vi "Plot Attributes.vi"(8 "error in (no error)":errorcluster, 10 "feature names":string[](array[string])=["feature1", "feature2", "feature3", "feature4"], 11 "appended array":refnum<vi>[](array[refnum])) -> (0 "error in (no error)":errorcluster)   [LabVIEW 2017, in "MachineLearning.lvlib"]
doc: "Replaces the plot names in the plot legend with the feature names for one or multiple waveform graphs."
uses:
  MachineLearning.lvlib
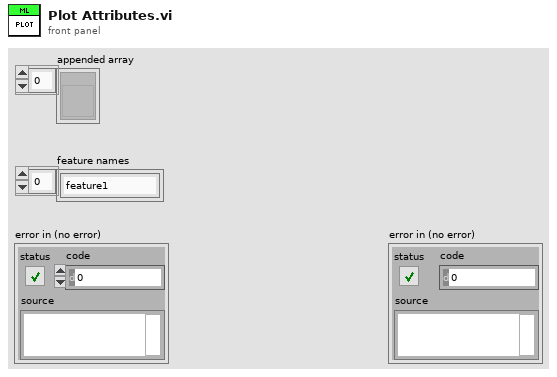
[diagram p1: front panel]
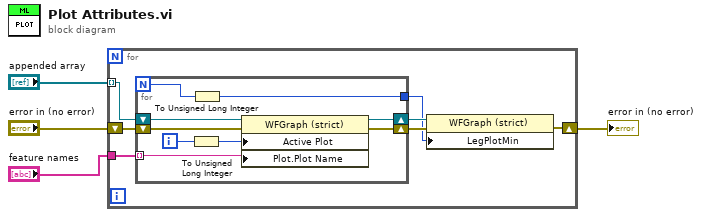
[diagram p0: block diagram]
diagram:
  n1 = for {
    tunnel: "appended array" -> [w7] mode=indexing
    tunnel: "feature names" -> [w11]
    shift-right: [w5] -> w1
    shift-left: "error in (no error)" -> [w10]
    n2 = for {
      N -> [w13]
      tunnel: w11 -> [w19] mode=indexing
      shift-right: [w18] -> w9
      shift-left: w10 -> [w20]
      shift-right: [w17] -> w8
      shift-left: w7 -> [w16]
      tunnel: [w12] -> w6
      i -> [w15]
      n3 = To Unsigned Long Integer(number=w15) -> (unsigned 32bit integer=w14:u32)
      n4 = To Unsigned Long Integer(number=w13) -> (unsigned 32bit integer=w12:u32)
      n5 = property class="WFGraph (strict)"(reference=w16, error in=w20, "Active Plot"=w14, "Plot.Plot Name"=w19) -> (reference out=w17:refnum<vi>, error out=w18:errorcluster)
    }
    n6 = property class="WFGraph (strict)"(reference=w8, error in=w9, "LegPlotMin"=w6) -> (error out=w5:errorcluster)  [unwired: 1 out]
  }
  "error in (no error)" <- w1
